vi "boolScalar.vi"(4 "Boolean":bool, 5 "msg in":string) -> (2 "msg out":string)   [LabVIEW 2013]
panel:
  out "unsigned byte array":u8[](array[numeric])
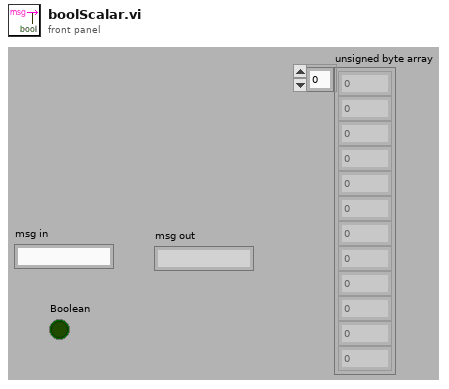
[diagram p1: front panel]
types:
  T1 = enum16{"big-endian, network order", "native, host order", "little-endian"}
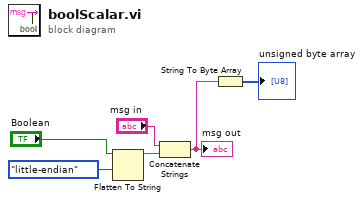
[diagram p0: block diagram]
diagram:
  n1 = Flatten To String(anything="Boolean", byte order (0:big-endian, network order)=T1."little-endian") -> (data string=w5:string)  [unwired: 2 in, 2 out]
  n2 = Concatenate Strings("msg in", w5) -> (w2:string)
  "msg out" <- w2
  n3 = String To Byte Array(string=w2) -> (unsigned byte array=→"unsigned byte array":u8[])
